vi "Set Emissivity.vi"(8 "error in (no error)":errorcluster, 10 "emissivity":u16, 11 "Temperature IR Bricklet in":refnum<class "Temperature IR Bricklet.lvclass">) -> (0 "error out":errorcluster, 3 "Temperature IR Bricklet out":refnum<class "Temperature IR Bricklet.lvclass">)   [LabVIEW 2011, in "Tinkerforge.lvlib" / "Temperature IR Bricklet.lvclass"]
doc: "This VI sets the emissivity. A integer value of 65535 is a emissivity of 1.0 and 0 is a emissivity of 0.0."
uses:
  Temperature IR Bricklet.lvclass
  Device/Device.lvclass
  IP Connection/IP Connection.lvclass
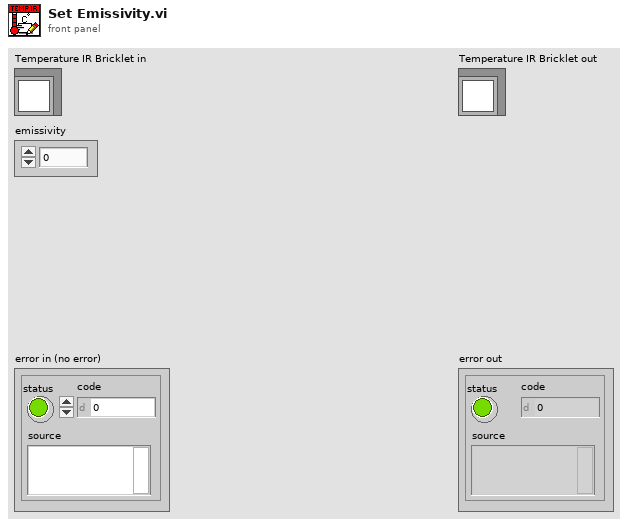
[diagram p1: front panel]
types:
  T1 = enum16{"big-endian, network order", "native, host order", "little-endian"}
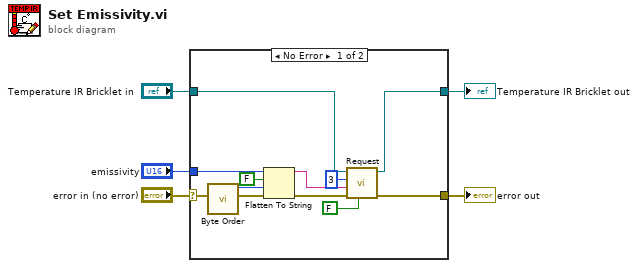
[diagram p0: block diagram]
diagram:
  n1 = case shown="No Error" "error in (no error)" {
    selector: "error in (no error)" -> [w11 w18]
    tunnel: [w12 w18] -> w4
    tunnel: [w15 w17] -> w2
    tunnel: "Temperature IR Bricklet in" -> [w16 w17]
    tunnel: "emissivity" -> [w8 _]
    frame No Error {
      n2 = call "Byte Order.vi"() -> ("byte order (2:little-endian)"=w6:T1)  [unwired: 11 in]
      n3 = Flatten To String(anything=w8, prepend array or string size? (T)=FALSE, byte order (0:big-endian, network order)=w6, error in (no error)=w11) -> (data string=w9:string, error out=w10:errorcluster)  [unwired: 1 out]
      n4 = call "Request.vi"("Response"=FALSE, "error in (no error)"=w10, "Data"=w9, "Function ID"=u8 3, "Device in"=w16) -> ("error out"=w12:errorcluster, "Device out"=w15:refnum<class "Temperature IR Bricklet.lvclass">)  [unwired: 2 in, 3 out]
    }
    frame Error {
    }
  }
  "error out" <- w4
  "Temperature IR Bricklet out" <- w2
